vi "SingleGUI_dualCH.vi"() -> ()   [LabVIEW 8.6]
uses:
  <vilib>/event_ctls.llb/lveventtype.ctl
  <vilib>/Utility/inputDevices.llb/mouseAcquire.vi
  <vilib>/Utility/inputDevices.llb/closeMouse.vi
panel:
  in  "EPI LED 3":bool
  in  "EPI LED 2":bool
  in  "Intensity 3":dbl(slide)
  in  "Intensity 2":dbl(slide)
  in  "Menu":string
  in  "Channel1":bool
  in  "Intensity":dbl(slide)
  in  "PMT2 ON":bool caption="PMT2"
  in  "High Voltage PMT / V 2":u16(slide) caption="High Voltage PMT2 / V"
  out "Gain 2":dbl caption="Gain 1" format="%^#_4g"
  in  "Pos [mm]":cluster{"x":dbl, "y":dbl} {"x" format="%.4f"; "y" format="%.4f"}
  in  "Stage control":enum32{"xy", "Setup", "Status"}(tab)
  in  "Stepsize [mm]":dbl(slide)
  in  "Cluster":T1
  in  "clockwise":bool
  in  "xy Angle":dbl
  out "scroll units^3":dbl
  out "Mouse inside?":T2
  out "scroll timed out":bool
  out "endGUI":bool
  in  "z[mm]":dbl(slide) scale format="%#.3f"
  in  "PMT Filter":sgl(ring) caption="filter.f1" items=["Split562", "Split495", "empty"]
  in  "Epi Filter":sgl(ring) caption="filter.f2" items=["emty", "empty"]
  in  "close":bool
  in  "PMT1 ON":bool caption="PMT1"
  in  "High Voltage PMT / V":u16(slide)
  out "Gain":dbl caption="Gain 1" format="%^#_4g"
  in  "stop 2":bool
  in  "continous":bool
  in  "EPI LED":bool
  in  "single":bool
  in  "Exposure (s)":dbl(slide) scale format="%#.3p"
  out "Image":T3(plugin-control)
  in  "Detector":u16(ring)
  out "Image Number":i32
  in  "Conversion Method":u32(ring) items=["Full Dynamic", "Given Range", "90% Dynamic", "Given Percent Range"]
  in  "Maximum Value":i32
  in  "Minimum Value":i32
  # "Colibri Laser Scanning                                                                                                                                                         TILL Photonics GmbH"
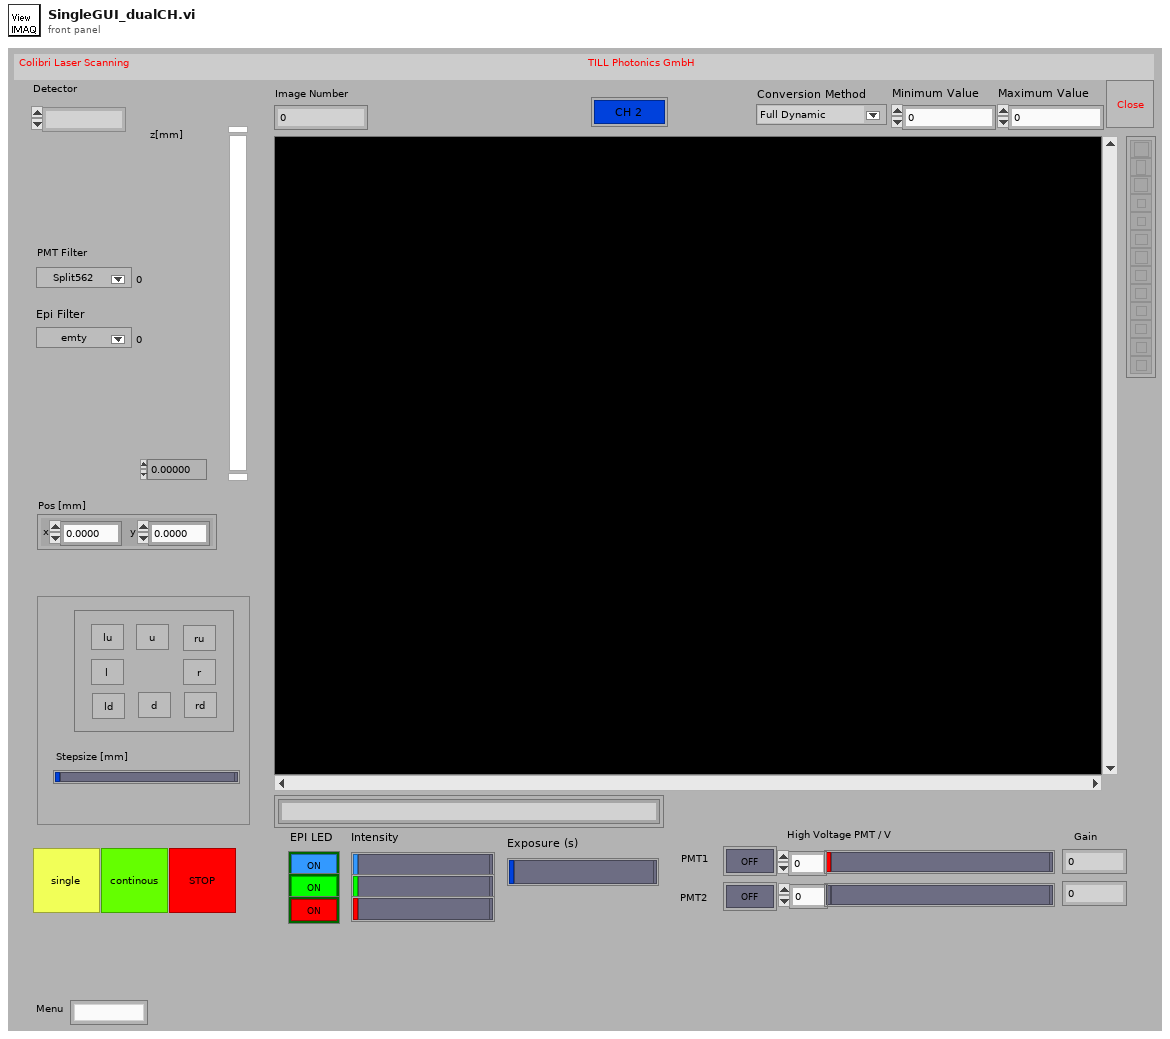
[diagram p1: front panel]
types:
  T1 = cluster{"r":bool, "ru":bool, "u":bool, "lu":bool, "l":bool, "ld":bool, "d":bool, "rd":bool}
  T2 = typedef "lveventtype.ctl" = enum32{"Null", "Timeout", "App Instance Close", "App Instance Close?", "Autoscale Range Change", "Cell Edit", "Cell Edit?", "Cursor Grab", "Cursor Grab?", "Cursor Move", "Cursor Release", "Data Change", "Direction Change", "Display State Change", "Drag Ended", "Drag Enter", "Drag Leave", "Drag Over", "Drag Source Update", "Drag Starting", "Drag Starting?", "Drop", "Exec State Change", "Key Down", "Key Down?", "Key Repeat", "Key Repeat?", "Key Up", "Listbox Double Click", "Menu Activation?", "Menu Selection (App)", "Menu Selection? (App)", "Menu Selection (User)", "Mouse Down", "Mouse Down?", "Mouse Enter", "Mouse Leave", "Mouse Move", "Mouse Up", "NI Security User Change (App)", "Pane Size", "Panel Close", "Panel Close?", "Panel Resize", "Plot Attribute Change", "Scale Range Change", "Shortcut Menu Activation?", "Shortcut Menu Selection (App)", "Shortcut Menu Selection? (App)", "Shortcut Menu Selection (User)", "Tree Double Click", "Tree Drag", "Tree Drag?", "Tree Drop", "Tree Drop?", "Tree Item Close", "Tree Item Close?", "Tree Item Open", "Tree Item Open?", "Value Change"}
  T3 = typedef "IMAQ Image.ctl" = refnum<image>
  T4 = enum16{"None/#Datasets", "Clear", "TagValueOf#", "AddValues", "ReadValue", "ChangeValue", "Get all"}
  T5 = enum16{"status", "createIMAQ", "getIMAQ", "getNumber", "deleteIMAQ", "deleteAll", "MemoryUsage", "GetAccess", "DecreaseAccess", "ActualIndex", "ElementToNumber"}
  T6 = cluster{"menu tag":string, "menu-vi":refnum<vi>}[]
  T7 = cluster{"Horizontal":i32, "Vertical":i32, "Scrolling":i32}
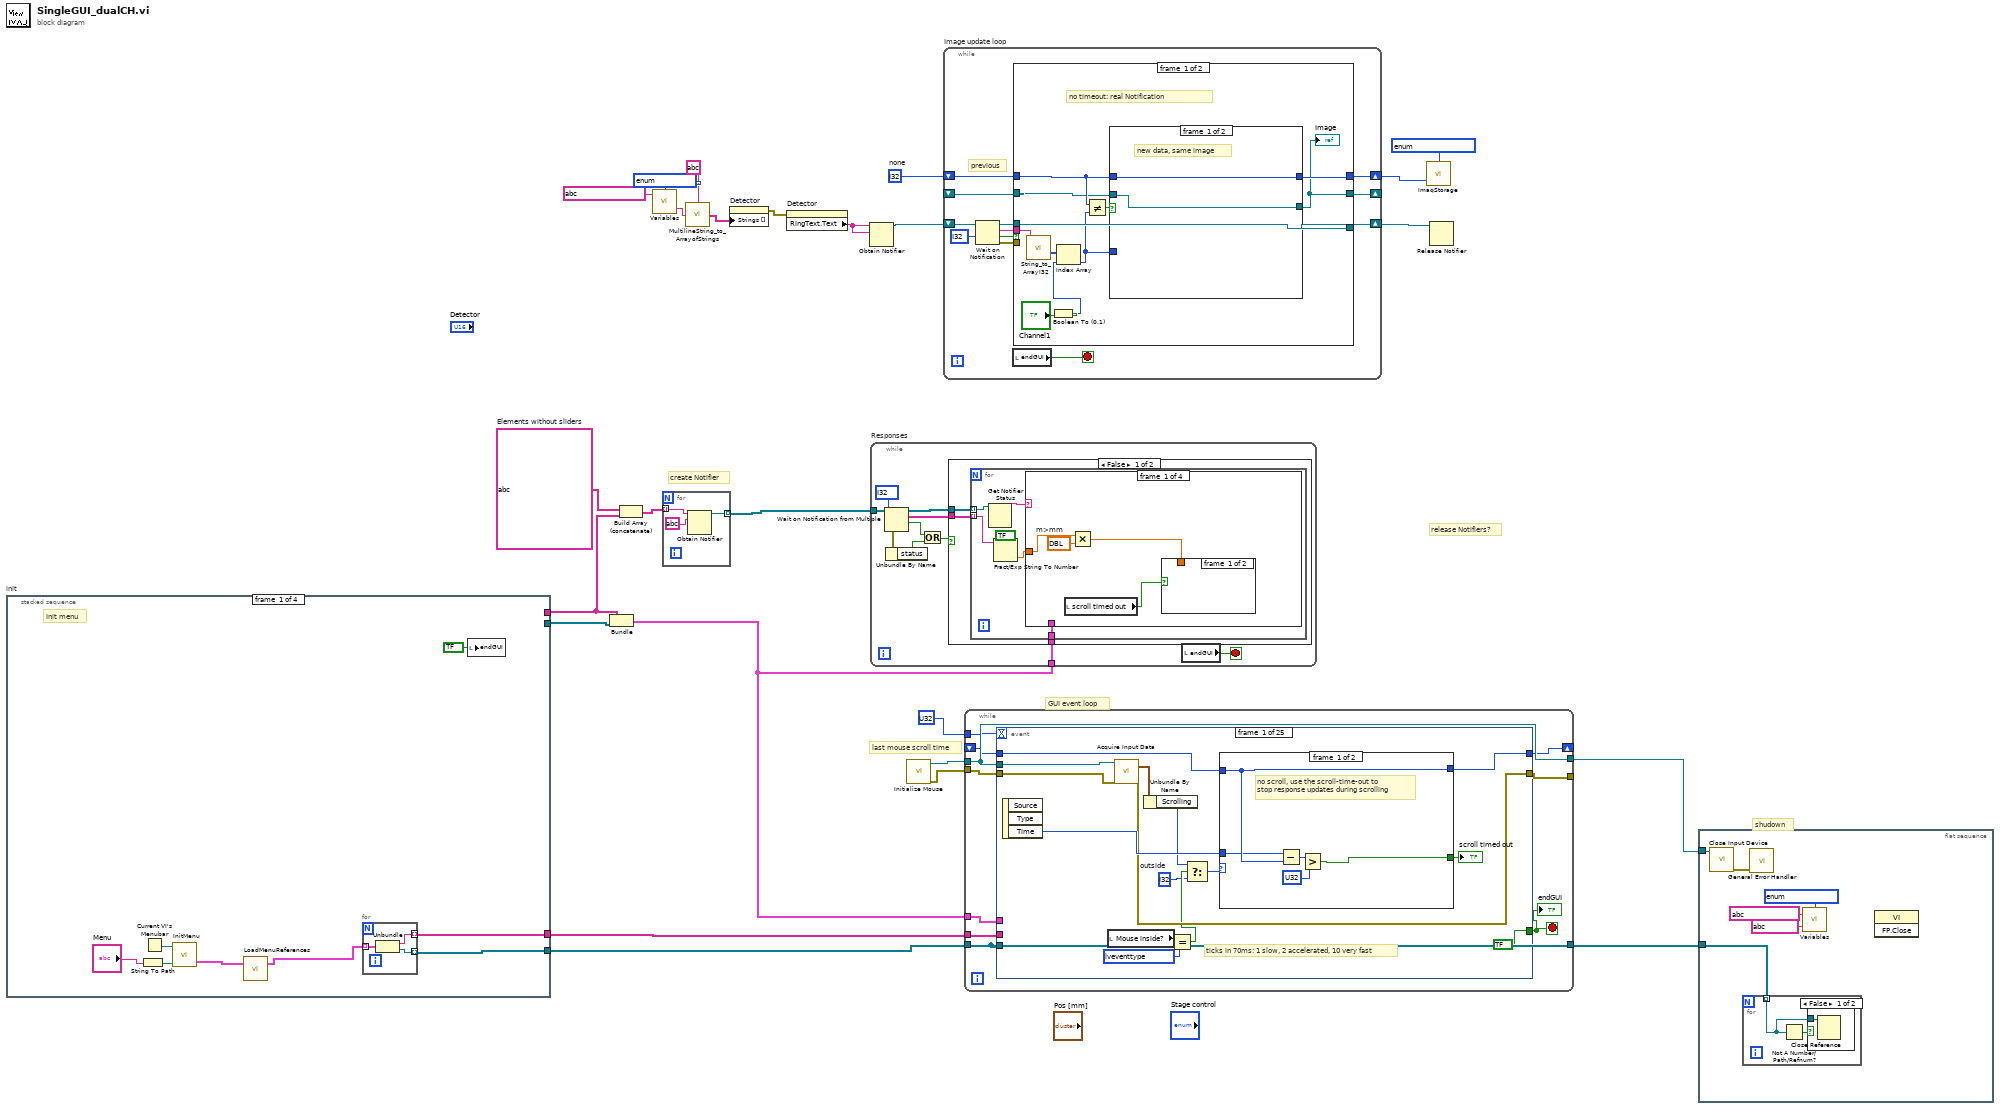
[diagram p0: block diagram]
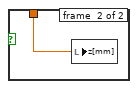
[diagram p3: hidden frame]
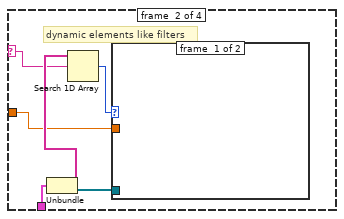
[diagram p4: hidden frame]
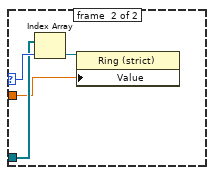
[diagram p5: hidden frame]
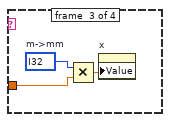
[diagram p6: hidden frame]
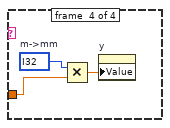
[diagram p7: hidden frame]
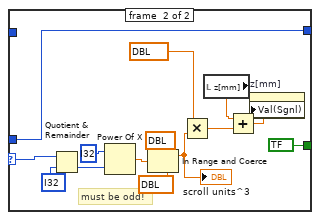
[diagram p9: hidden frame]
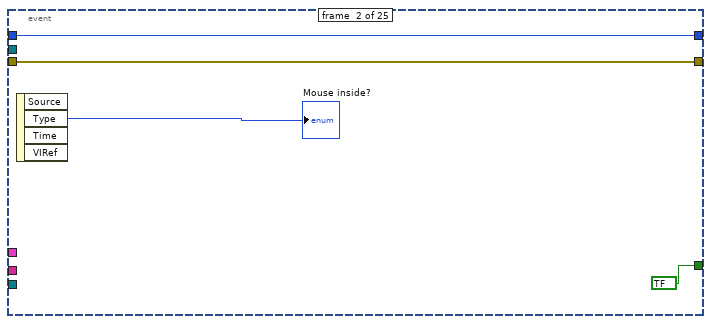
[diagram p10: hidden frame]
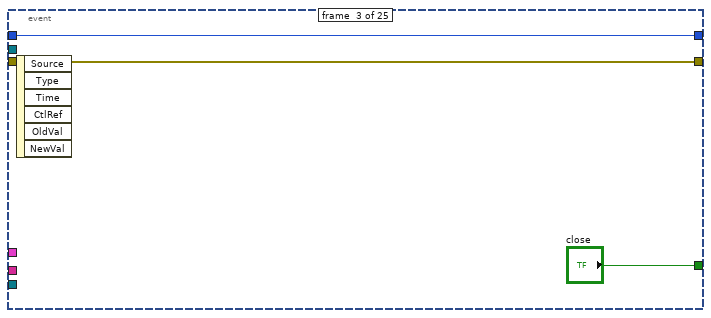
[diagram p11: hidden frame]
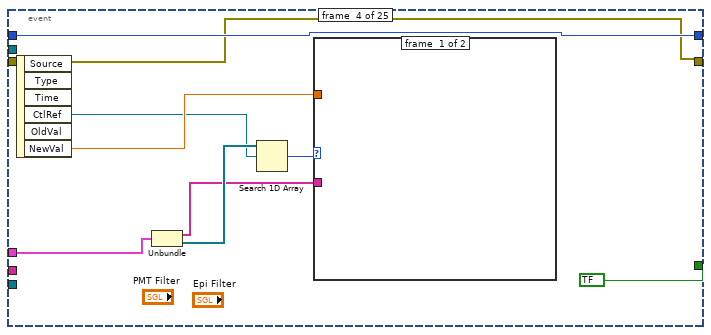
[diagram p12: hidden frame]
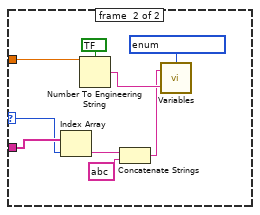
[diagram p13: hidden frame]
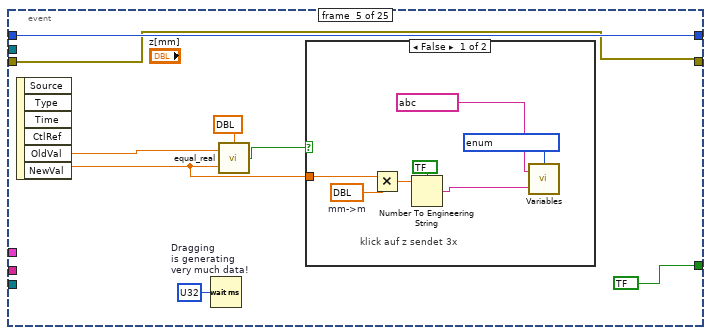
[diagram p14: hidden frame]
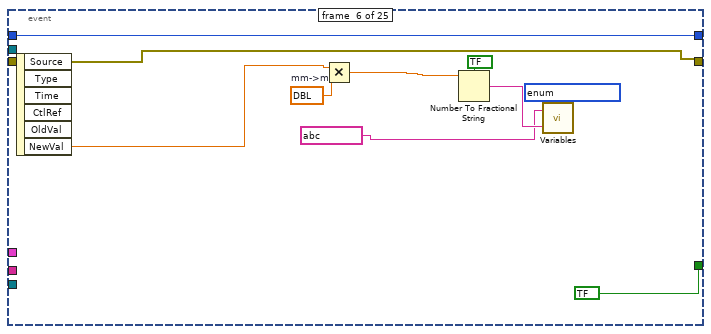
[diagram p16: hidden frame]
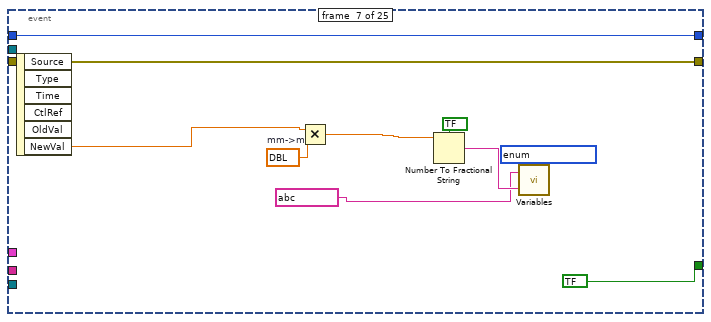
[diagram p17: hidden frame]
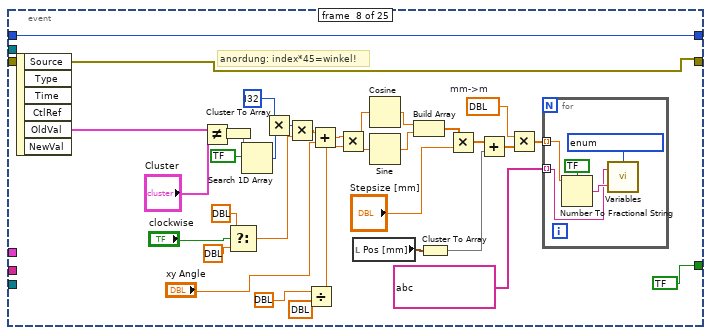
[diagram p18: hidden frame]
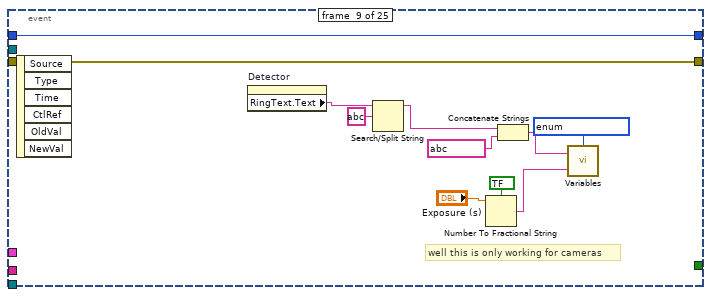
[diagram p19: hidden frame]
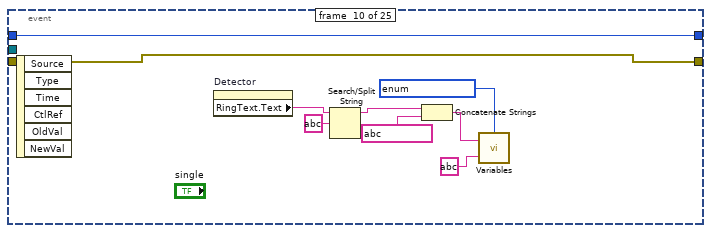
[diagram p20: hidden frame]
diagram:
  w13 = string[] ?  # Elements without sliders
  w22 = i32 ?  # none
  # "shudown"
  # "last mouse scroll time"
  # "release Notifiers?"
  # "create Notifier"
  # "GUI event loop"
  n1 = stacked-sequence "init" {
    tunnel: [_ w41 _ _] -> w11
    tunnel: [_ w40 _ _] -> w9
    tunnel: [w27 _ _ _] -> w4
    tunnel: [w26 _ _ _] -> w3
    frame #0 {
      # "Init menu"
      n2 = String To Path(string="Menu") -> (path=w30:path)
      n3 = Current VI's Menubar() -> (w32:refnum<k9>)
      n4 = call "InitMenu.vi"("menu-ini"=w30, "menubar"=w32) -> ("Menu-VI"=w31:cluster{"item tag":string, "vi-Path":path}[])  [unwired: 1 out]
      n5 = call "LoadMenuReferences.vi"("Menu-VI"=w31) -> ("Menu"=w28:T6)  [unwired: 1 in, 1 out]
      n6 = for {
        tunnel: w28 -> [w36] mode=indexing
        tunnel: [w35] -> w27 mode=indexing
        tunnel: [w34] -> w26 mode=indexing
        n7 = Unbundle(w36) -> ("menu tag"=w35:string, "menu-vi"=w34:refnum<vi>)
      }
      n8 = local write "endGUI"(bool ? ("stop 2")) -> ()
    }
    frame #1 {
      # "Init filter slider controls"
      n9 = call "Variables.vi"("Tag in"=string ?, "Command"=T4 ?) -> ("value out"=w43:string)  [unwired: 1 in, 2 out]
      n10 = call "MultilineString_to_ArrayofStrings.vi"("String 1"=w43, "NewLineString"=string ?) -> ("String Array"=w41:string[])
      n11 = control-ref of="Epi Filter"() -> (w39:refnum<vi>)
      n12 = control-ref of="PMT Filter"() -> (w38:refnum<vi>)
      n13 = Build Array(w38, w39) -> (w37:refnum<vi>[])
      n14 = for {
        tunnel: w41 -> [w49] mode=indexing
        tunnel: w37 -> [w47] mode=indexing
        tunnel: [w46] -> w40 mode=indexing
        n15 = Concatenate Strings(w49, string ? ("string")) -> (w50:string)
        n16 = call "Variables.vi"("Tag in"=w50, "Command"=T4 ?) -> ("value out"=w54:string)  [unwired: 1 in, 2 out]
        n17 = call "MultilineString_to_ArrayofStrings.vi"("String 1"=w54, "NewLineString"=string ?) -> ("String Array"=w53:string[])
        n18 = for {
          tunnel: w53 -> [w63] mode=indexing
          tunnel: [w58] -> w52 mode=indexing
          n19 = call "SplitAtLast.vi"("search char"=string ?, "In-String"=w63) -> ("end"=w61:string, "Front (default)"=w60:string)
          n20 = Fract/Exp String To Number(use system decimal point (T)=bool ?, string=w61) -> (number=w59:dbl)  [unwired: 3 out]
          n21 = Bundle("Front (default)"=w60, w59) -> (w58:cluster{"Front (default)":string, dbl})  [unwired: 1 out]
        }
        n22 = property on="Property Node" class="Ring (strict)"(reference=w47, "StringsAndValues[]"=w52, "Visible"=bool ?, "Caption.Text"=w49) -> (reference out=w46:refnum<vi>)  [unwired: 1 in, 1 out]
      }
    }
    frame #2 {
      # "it would be good to Read/update all elements\nbut this is usually done by \"update\" to the .set variables after the return Notifiers are listening\nhere just z is updated"
      n23 = call "Variables.vi"("Tag in"=string ?, "Command"=T4 ?) -> ("value out"=w67:string)  [unwired: 1 in, 2 out]
      n24 = Fract/Exp String To Number(use system decimal point (T)=bool ?, string=w67) -> (number=w66:dbl)  [unwired: 3 out]
      n25 = Multiply(x=dbl ?, y=w66) -> (x*y=w65:dbl)
      n26 = local write "z[mm]"(w65) -> ()
    }
    frame #3 {
      n27 = property on="Image" class="ImageControl"() -> ("16-bit Display Conversion Method"=w71:u32)  [unwired: 2 in, 2 out]
      n28 = local write "Conversion Method"(w71) -> ()
    }
  }
  n29 = Bundle("String Array"=w11, w9) -> (w10:cluster{"String Array":string[], refnum<vi>[]})  [unwired: 1 out]
  n30 = Build Array (concatenate)(w13, w11) -> (w12:string[])
  n31 = call "Variables.vi"("Tag in"=string ?, "Command"=T4 ?) -> ("value out"=w17:string)  [unwired: 1 in, 2 out]
  n32 = for {
    tunnel: w12 -> [w73] mode=indexing
    tunnel: [w74] -> w8 mode=indexing
    n33 = Obtain Notifier(name (unnamed)=w73, notification data type=string ?) -> (notifier out=w74:refnum<notifier>)  [unwired: 2 in, 2 out]
  }
  n34 = call "MultilineString_to_ArrayofStrings.vi"("String 1"=w17, "NewLineString"=string ?) -> ("String Array"=w15:string[])
  n35 = property on="Detector" class="Ring (strict)"("Strings []"=w15) -> (error out=w14:errorcluster)  [unwired: 2 in, 1 out]
  n36 = property on="Detector" class="Ring (strict)"(error in=w14) -> ("RingText.Text"=w23:string)  [unwired: 1 in, 2 out]
  n37 = Obtain Notifier(name (unnamed)=w23, notification data type=w23) -> (notifier out=w25:refnum<notifier>)  [unwired: 2 in, 2 out]
  n38 = while "Responses" {
    tunnel: w8 -> [w84]
    tunnel: w10 -> [w76]
    stop <- w75 stop-if-true
    n39 = Wait on Notification from Multiple(0:w84, 2:i32 ? ("timeout in ms (-1)")) -> (8:w79:refnum<notifier>[], 9:w78:string[], 10:w80:bool, 11:w82:errorcluster)  [unwired: 1 in, 1 out]
    n40 = Unbundle By Name(w82) -> ("status"=w81:bool)
    n41 = Or(x=w80, y=w81) -> (x .or. y?=w77:bool)
    n42 = case shown="False" w77 {
      tunnel: w79 -> [w87 _]
      tunnel: w78 -> [w86 _]
      tunnel: w76 -> [w85 _]
      frame #0 {
        n43 = for {
          tunnel: w87 -> [w93] mode=indexing
          tunnel: w86 -> [w91] mode=indexing
          tunnel: w85 -> [w88]
          n44 = Get Notifier Status(notifier=w93) -> (notifier name=w92:string)  [unwired: 1 in, 4 out]
          n45 = Fract/Exp String To Number(use system decimal point (T)=bool ?, string=w91) -> (number=w89:dbl)  [unwired: 3 out]
          n46 = case shown="\"filter.f1\", Default" w92 {
            selector: w92 -> [_ w101 _ _]
            tunnel: w89 -> [w97 w99 w110 w114]
            tunnel: w88 -> [_ w104 _ _]
            frame #0 {
              w95 = dbl ?  # m>mm
              n47 = local read "scroll timed out"() -> (w94:bool)
              n48 = Multiply(x=w97, y=w95) -> (x*y=w96:dbl)
              n49 = case shown="True" w94 {
                tunnel: w96 -> [_ w98]
                frame #0 {
                }
                frame #1 {
                  n50 = local write "z[mm]"(w98) -> ()
                }
              }
            }
            frame #1 {
              # "dynamic elements like filters"
              n51 = Unbundle(w104) -> ("String Array"=w102:string[], w103:refnum<vi>[])
              n52 = Search 1D Array(1D array=w102, element=w101) -> (index of element=w100:i32)  [unwired: 1 out]
              n53 = case shown="0.." w100 {
                selector: w100 -> [_ w108]
                tunnel: w103 -> [_ w107]
                tunnel: w99 -> [_ w105]
                frame #0 {
                }
                frame #1 {
                  n54 = Index Array(array=w107, index=w108) -> (element=w106:refnum<vi>)
                  n55 = property on="Property Node" class="Ring (strict)"(reference=w106, "Value"=w105) -> ()  [unwired: 1 in, 2 out]
                }
              }
            }
            frame #2 {
              w111 = i32 ?  # m->mm
              n56 = Multiply(x=w111, y=w110) -> (x*y=w109:dbl)
              n57 = property on="x" class="DigNum (strict)"("Value"=w109) -> ()  [unwired: 2 in, 2 out]
            }
            frame #3 {
              w113 = i32 ?  # m->mm
              n58 = Multiply(x=w113, y=w114) -> (x*y=w112:dbl)
              n59 = property on="y" class="DigNum (strict)"("Value"=w112) -> ()  [unwired: 2 in, 2 out]
            }
          }
        }
      }
      frame #1 {
        # "err or timeout"
      }
    }
    n60 = local read "endGUI"() -> (w75:bool)
  }
  n61 = call <vilib>:"Initialize Mouse.vi"() -> ("error out"=w6:errorcluster, "device ID"=w7:refnum<k1>)  [unwired: 1 in, 9 out]
  n62 = while "Image update loop" {
    shift-right: [w124] -> w21
    shift-left: w22 -> [w125]
    shift-right: [w119] -> w24
    shift-left: w25 -> [w126]
    shift-right: [w118] -> _
    shift-left: _ -> [w117]
    stop <- w116 stop-if-true
    # "previous"
    n63 = Wait on Notification(notifier=w126, timeout in ms (-1)=i32 ?) -> (notifier out=w120:refnum<notifier>, notification=w115:string, timed out?=w122:bool, error out=w123:errorcluster)  [unwired: 1 in, 1 out]
    n64 = local read "endGUI"() -> (w116:bool)
    n65 = case shown="True" w122 {
      tunnel: w115 -> [w131 _]
      tunnel: w125 -> [w136 w152]
      tunnel: [w133 w152] -> w124
      tunnel: w123 -> [_ _]
      tunnel: w120 -> [w137 w151]
      tunnel: [w137 w147] -> w119
      tunnel: [w132 w145] -> w118
      tunnel: w117 -> [w134 w145]
      frame #0 {
        # "no timeout: real Notification"
        n66 = call "String_to_ArrayI32.vi"("String"=w131) -> ("ArrayI32"=w130:i32[])  [unwired: 1 in]
        n67 = Boolean To (0,1)(Boolean="Channel1") -> (0, 1=w127:i16)
        n68 = Index Array(array=w130, index=w127) -> (element=w129:i32)
        n69 = Not Equal?(x=w136, y=w129) -> (x != y?=w135:bool)
        n70 = case shown="True" w135 {
          tunnel: [w139 w144] -> w132
          tunnel: w129 -> [_ w140]
          tunnel: w136 -> [w138 w143]
          tunnel: w134 -> [w139 _]
          tunnel: [w138 w140] -> w133
          frame #0 {
            # "new data, same image"
          }
          frame #1 {
            # "only valid if\nstill in memory!"
            # "new image"
            n71 = call "ImaqStorage.vi"("Number"=w143, "Command"=T5 ?) -> ()  [unwired: 1 in, 2 out]
            n72 = call "ImaqStorage.vi"("Number"=w140, "Command"=T5 ?) -> ("IMAQ out"=w144:T3)  [unwired: 1 in, 1 out]
            "Image Number" <- w140
          }
        }
        "Image" <- w132
      }
      frame #1 {
        # "time out\ngood for checking the stop button\nis there a new detektor?"
        n73 = property on="Detector" class="Ring (strict)"() -> ("RingText.Text"=w146:string)  [unwired: 2 in, 2 out]
        n74 = Get Notifier Status(notifier=w151) -> (notifier out=w148:refnum<notifier>, notifier name=w150:string)  [unwired: 1 in, 3 out]
        n75 = Not Equal?(x=w146, y=w150) -> (x != y?=w149:bool)
        n76 = case shown="True" w149 {
          tunnel: w148 -> [w153 w156]
          tunnel: [w153 w155] -> w147
          tunnel: w146 -> [_ w154]
          frame #0 {
            # "same as before"
          }
          frame #1 {
            n77 = Release Notifier(notifier=w156) -> ()  [unwired: 1 in, 4 out]
            n78 = Obtain Notifier(name (unnamed)=w154, notification data type=w154) -> (notifier out=w155:refnum<notifier>)  [unwired: 2 in, 2 out]
          }
        }
      }
    }
  }
  n79 = while {
    tunnel: w10 -> [w166]
    tunnel: w7 -> [w165]
    tunnel: [w165] -> w2
    tunnel: w6 -> [w164]
    tunnel: [w163] -> _
    shift-right: [w161] -> _
    shift-left: _ -> [w162]
    tunnel: u32 ? ("milliseconds to wait") -> [w159]
    tunnel: w4 -> [w158]
    tunnel: w3 -> [w157]
    tunnel: [w157] -> w1
    stop <- w160 stop-if-true
    n80 = event shown="[23] Menu Selection (User)" {
      selector: _ -> [_ _ _ _ _ _ _ _ _ _ _ _ _ _ _ _ _ _ _ _ _ _ _ _ _]
      dyn-events: _ -> [_ _ _ _ _ _ _ _ _ _ _ _ _ _ _ _ _ _ _ _ _ _ _ _ _]
      timeout: w159 -> [_ _ _ _ _ _ _ _ _ _ _ _ _ _ _ _ _ _ _ _ _ _ _ _ _]
      tunnel: [bool ? ("stop") bool ? ("stop") "close" bool ? bool ? bool ? bool ? ("stop") bool ? ("stop") _ _ _ _ _ _ _ _ _ _ bool ? ("stop") bool ? ("stop") _ _ _ w432 w445] -> w160
      tunnel: w166 -> [_ _ _ w214 _ _ _ _ _ _ _ _ _ _ _ _ _ _ _ _ _ _ _ _ _]
      tunnel: w165 -> [w181 _ _ _ _ _ _ _ _ _ _ _ _ _ _ _ _ _ _ _ _ _ _ _ _]
      tunnel: w164 -> [w180 w201 w205 w208 w226 w242 w251 w261 w302 w313 w319 w327 w335 w346 w355 w361 w366 w375 w385 w397 w410 w417 w424 _ _]
      tunnel: [w173 w201 w205 w208 w226 w242 w251 w261 w302 w313 w319 w327 w335 w346 w355 w361 w366 w375 w385 w397 w410 w417 w424 _ _] -> w163
      tunnel: w162 -> [w177 w202 w206 w209 w227 w241 w252 w262 w303 w314 w320 w328 w336 w347 w356 w362 w367 w376 w386 w398 w416 w423 w430 w431 w444]
      tunnel: [w178 w202 w206 w209 w227 w241 w252 w262 w303 w314 w320 w328 w336 w347 w356 w362 w367 w376 w386 w398 w416 w423 w430 w431 w444] -> w161
      tunnel: w158 -> [_ _ _ _ _ _ _ _ _ _ _ _ _ _ _ _ _ _ _ _ _ _ _ w434 _]
      tunnel: w157 -> [_ _ _ _ _ _ _ _ _ _ _ _ _ _ _ _ _ _ _ _ _ _ _ w433 _]
      event #0 {
        w167 = i32 ?  # outside
        # "ticks in 70ms: 1 slow, 2 accelerated, 10 very fast"
        n81 = event-data() -> ("Time"=w176:u32)  [unwired: 3 out]
        n82 = local read "Mouse inside?"() -> (w172:T2)
        n83 = call-poly <vilib>:"Acquire Input Data.vi"("device ID"=w181, "error in (no error)"=w180) -> ("axis info"=w179:T7, "error out"=w173:errorcluster)  [unwired: 1 in, 15 out]
        n84 = Unbundle By Name(w179) -> ("Scrolling"=w169:i32)
        n85 = Equal?(x=w172, y=T2 ? ("Type")) -> (x = y?=w170:bool)
        n86 = Select(t=w169, s=w170, f=w167) -> (s? t:f=w168:i32)
        n87 = case shown="1, Default" w168 {
          selector: w168 -> [_ w196]
          tunnel: w177 -> [w186 _]
          tunnel: [w186 w197] -> w178
          tunnel: w176 -> [w183 w197]
          tunnel: [w182 bool ?] -> w174
          frame #0 {
            # "no scroll, use the scroll-time-out to\nstop response updates during scrolling"
            n88 = Subtract(x=w183, y=w186) -> (x-y=w185:u32)
            n89 = Greater?(x=w185, y=u32 ?) -> (0:w182:bool)
          }
          frame #1 {
            # "must be odd!"
            n90 = Quotient & Remainder(x=w196, y=i32 ?) -> (floor(x/y)=w194:i32)  [unwired: 1 out]
            n91 = Power Of X(1:w194, 2:i32 ? ("y")) -> (0:w192:dbl)
            n92 = In Range and Coerce(upper limit=dbl ?, x=w192, lower limit=dbl ?) -> (coerced(x)=w191:dbl)  [unwired: 1 out]
            "scroll units^3" <- w191
            n93 = Multiply(x=dbl ? ("min.step"), y=w191) -> (x*y=w200:dbl)
            n94 = local read "z[mm]"() -> (w199:dbl)
            n95 = Add(x=w199, y=w200) -> (x+y=w198:dbl)
            n96 = property on="z[mm]" class="Slide (strict)"("Val(Sgnl)"=w198) -> ()  [unwired: 2 in, 2 out]
          }
        }
        "scroll timed out" <- w174
      }
      event #1 {
        n97 = event-data() -> ("Type"=→"Mouse inside?":T2)  [unwired: 4 out]
      }
      event #2 {
        n98 = event-data() -> ()  [unwired: 7 out]
      }
      event #3 {
        n99 = event-data() -> ("CtlRef"=w212:refnum<vi>, "NewVal"=w216:sgl)  [unwired: 5 out]
        n100 = Unbundle(w214) -> ("String Array"=w210:string[], w213:refnum<vi>[])
        n101 = Search 1D Array(1D array=w213, element=w212) -> (index of element=w211:i32)  [unwired: 1 out]
        n102 = case shown="0.." w211 {
          selector: w211 -> [_ w220]
          tunnel: w216 -> [_ w225]
          tunnel: w210 -> [_ w221]
          frame #0 {
          }
          frame #1 {
            n103 = Index Array(array=w221, index=w220) -> (element=w219:string)
            n104 = Number To Engineering String(1:bool ? ("use system decimal point (T)"), 4:w225) -> (0:w224:string)  [unwired: 2 out]
            n105 = Concatenate Strings(w219, string ? ("string")) -> (w218:string)
            n106 = call "Variables.vi"("value"=w224, "Tag in"=w218, "Command"=T4 ?) -> ()  [unwired: 3 out]
          }
        }
      }
      event #4 {
        w232 = u32 ?  # Dragging is generating very much data!
        n107 = event-data() -> ("OldVal"=w231:dbl, "NewVal"=w230:dbl)  [unwired: 5 out]
        n108 = Wait (ms)(milliseconds to wait=w232) -> ()  [unwired: 1 out]
        n109 = call "equal_real.vi"("max rel deviation"=dbl ?, "b"=w230, "a"=w231) -> ("Equal"=w229:bool)
        n110 = case shown="False" w229 {
          tunnel: w230 -> [w235 _]
          frame #0 {
            w240 = dbl ?  # mm->m
            # "klick auf z sendet 3x"
            n111 = Multiply(x=w235, y=w240) -> (x*y=w239:dbl)
            n112 = Number To Engineering String(1:bool ? ("use system decimal point (T)"), 4:w239) -> (0:w237:string)  [unwired: 2 out]
            n113 = call "Variables.vi"("value"=w237, "Tag in"=string ?, "Command"=T4 ?) -> ()  [unwired: 3 out]
          }
          frame #1 {
          }
        }
      }
      event #5 {
        w249 = dbl ?  # mm->m
        n114 = event-data() -> ("NewVal"=w247:dbl)  [unwired: 6 out]
        n115 = Multiply(x=w247, y=w249) -> (x*y=w250:dbl)
        n116 = Number To Fractional String(use system decimal point (T)=bool ?, number=w250) -> (F-format string=w245:string)  [unwired: 2 out]
        n117 = call "Variables.vi"("value"=w245, "Tag in"=string ? ("Tag"), "Command"=T4 ?) -> ()  [unwired: 3 out]
      }
      event #6 {
        w259 = dbl ?  # mm->m
        n118 = event-data() -> ("NewVal"=w254:dbl)  [unwired: 6 out]
        n119 = Multiply(x=w254, y=w259) -> (x*y=w260:dbl)
        n120 = Number To Fractional String(use system decimal point (T)=bool ?, number=w260) -> (F-format string=w257:string)  [unwired: 2 out]
        n121 = call "Variables.vi"("value"=w257, "Tag in"=string ? ("Tag"), "Command"=T4 ?) -> ()  [unwired: 3 out]
      }
      event #7 {
        w277 = dbl ?  # mm->m
        # "anordung: index*45=winkel!"
        n122 = event-data() -> ("OldVal"=w293:T1)  [unwired: 6 out]
        n123 = Not Equal?(x=w293, y="Cluster") -> (x != y?=w292:T1)
        n124 = Cluster To Array(cluster=w292) -> (array=w291:bool[])
        n125 = Select(t=dbl ?, s="clockwise", f=dbl ?) -> (s? t:f=w266:dbl)
        n126 = Search 1D Array(1D array=w291, element=bool ? ("Element")) -> (index of element=w289:i32)  [unwired: 1 out]
        n127 = Multiply(x=i32 ?, y=w289) -> (x*y=w288:i32)
        n128 = Multiply(x=w288, y=w266) -> (x*y=w267:dbl)
        n129 = Divide(x=dbl ?, y=dbl ?) -> (x/y=w268:dbl)
        n130 = Add(x=w267, y="xy Angle") -> (x+y=w265:dbl)
        n131 = Multiply(x=w265, y=w268) -> (x*y=w275:dbl)
        n132 = local read "Pos [mm]"() -> (w282:cluster{"x":dbl, "y":dbl})
        n133 = Cosine(x=w275) -> (cos(x)=w285:dbl)
        n134 = Sine(x=w275) -> (sin(x)=w284:dbl)
        n135 = Build Array(w285, w284) -> (w283:dbl[])
        n136 = Cluster To Array(cluster=w282) -> (array=w281:dbl[])
        n137 = Multiply(x=w283, y="Stepsize [mm]") -> (x*y=w286:dbl[])
        n138 = Add(x=w286, y=w281) -> (x+y=w279:dbl[])
        n139 = Multiply(x=w277, y=w279) -> (x*y=w278:dbl[])
        n140 = for {
          tunnel: w278 -> [w294] mode=indexing
          tunnel: string[] ? -> [w295] mode=indexing
          n141 = Number To Fractional String(use system decimal point (T)=bool ?, number=w294) -> (F-format string=w298:string)  [unwired: 2 out]
          n142 = call "Variables.vi"("value"=w298, "Tag in"=w295, "Command"=T4 ?) -> ()  [unwired: 3 out]
        }
      }
      event #8 {
        # "well this is only working for cameras"
        n143 = event-data() -> ()  [unwired: 7 out]
        n144 = property on="Detector" class="Ring (strict)"() -> ("RingText.Text"=w300:string)  [unwired: 2 in, 2 out]
        n145 = Search/Split String(string=w300, search string/char (-)=string ? ("Nach String/Zeichen suchen (-)")) -> (substring before match=w299:string)  [unwired: 3 out]
        n146 = Number To Fractional String(use system decimal point (T)=bool ?, number="Exposure (s)") -> (F-format string=w306:string)  [unwired: 2 out]
        n147 = Concatenate Strings(w299, string ? ("Tag in")) -> (w309:string)
        n148 = call "Variables.vi"("value"=w306, "Tag in"=w309, "Command"=T4 ?) -> ()  [unwired: 3 out]
      }
      event #9 {
        n149 = event-data() -> ()  [unwired: 7 out]
        n150 = property on="Detector" class="Ring (strict)"() -> ("RingText.Text"=w311:string)  [unwired: 2 in, 2 out]
        n151 = Search/Split String(string=w311, search string/char (-)=string ? ("Nach String/Zeichen suchen (-)")) -> (substring before match=w310:string)  [unwired: 3 out]
        n152 = Concatenate Strings(w310, string ? ("notification")) -> (w317:string)
        n153 = call "Variables.vi"("value"=string ? ("notification"), "Tag in"=w317, "Command"=T4 ?) -> ()  [unwired: 3 out]
      }
      event #10 {
        n154 = event-data() -> ()  [unwired: 7 out]
        n155 = Select(t=string ? ("value"), s="EPI LED", f=string ?) -> (s? t:f=w325:string)
        n156 = call "Variables.vi"("value"=w325, "Tag in"=string ?, "Command"=T4 ?) -> ()  [unwired: 3 out]
      }
      event #11 {
        n157 = event-data() -> ()  [unwired: 7 out]
        n158 = Select(t=string ? ("value"), s="EPI LED 3", f=string ?) -> (s? t:f=w333:string)
        n159 = call "Variables.vi"("value"=w333, "Tag in"=string ?, "Command"=T4 ?) -> ()  [unwired: 3 out]
      }
      event #12 {
        n160 = event-data() -> ()  [unwired: 7 out]
        n161 = Select(t=string ? ("value"), s="EPI LED 2", f=string ?) -> (s? t:f=w341:string)
        n162 = call "Variables.vi"("value"=w341, "Tag in"=string ?, "Command"=T4 ?) -> ()  [unwired: 3 out]
      }
      event #13 {
        n163 = event-data() -> ()  [unwired: 7 out]
        n164 = property on="Detector" class="Ring (strict)"() -> ("RingText.Text"=w344:string)  [unwired: 2 in, 2 out]
        n165 = Search/Split String(string=w344, search string/char (-)=string ? ("Nach String/Zeichen suchen (-)")) -> (substring before match=w343:string)  [unwired: 3 out]
        n166 = Concatenate Strings(w343, string ? ("notification")) -> (w351:string)
        n167 = call "Variables.vi"("value"=string ? ("notification"), "Tag in"=w351, "Command"=T4 ?) -> ()  [unwired: 3 out]
      }
      event #14 {
        n168 = event-data() -> ()  [unwired: 7 out]
        n169 = property on="Detector" class="Ring (strict)"() -> ("RingText.Text"=w353:string)  [unwired: 2 in, 2 out]
        n170 = Search/Split String(string=w353, search string/char (-)=string ? ("Nach String/Zeichen suchen (-)")) -> (substring before match=w352:string)  [unwired: 3 out]
        n171 = Concatenate Strings(w352, string ? ("notification")) -> (w359:string)
        n172 = call "Variables.vi"("value"=string ? ("notification"), "Tag in"=w359, "Command"=T4 ?) -> ()  [unwired: 3 out]
      }
      event #15 {
        n173 = event-data() -> ()  [unwired: 7 out]
        n174 = property on="Image" class="ImageControl"("16-bit Display Conversion Method"="Conversion Method", "16-bit Display Maximum Value"="Maximum Value", "16-bit Display Minimum Value"="Minimum Value") -> ()  [unwired: 2 in, 2 out]
      }
      event #16 {
        n175 = event-data() -> ("NewVal"=w368:u16)  [unwired: 6 out]
        n176 = call "PMT-Gain.vi"("Volt"=w368) -> ("Gain"=→"Gain":dbl)
        n177 = local read "PMT1 ON"() -> (w369:bool)
        n178 = case shown="True" w369 {
          tunnel: w368 -> [_ w374]
          frame #0 {
          }
          frame #1 {
            n179 = Number To Decimal String(number=w374) -> (decimal integer string=w371:string)  [unwired: 1 out]
            n180 = call "Variables.vi"("value"=w371, "Tag in"=string ?, "Command"=T4 ?) -> ()  [unwired: 3 out]
          }
        }
      }
      event #17 {
        n181 = event-data() -> ("NewVal"=w377:u16)  [unwired: 6 out]
        n182 = call "PMT-Gain.vi"("Volt"=w377) -> ("Gain"=→"Gain 2":dbl)
        n183 = local read "PMT2 ON"() -> (w378:bool)
        n184 = case shown="True" w378 {
          tunnel: w377 -> [_ w383]
          frame #0 {
          }
          frame #1 {
            n185 = Number To Decimal String(number=w383) -> (decimal integer string=w380:string)  [unwired: 1 out]
            n186 = call "Variables.vi"("value"=w380, "Tag in"=string ?, "Command"=T4 ?) -> ()  [unwired: 3 out]
          }
        }
      }
      event #18 {
        n187 = event-data() -> ()  [unwired: 7 out]
        n188 = case shown="True" "PMT1 ON" {
          tunnel: [string ? w395] -> w390
          tunnel: [u8 ? ("Disabled") u8 ? ("Disabled")] -> w391
          frame #0 {
            # "send 0"
          }
          frame #1 {
            # "send"
            n189 = Number To Decimal String(number="High Voltage PMT / V") -> (decimal integer string=w395:string)  [unwired: 1 out]
          }
        }
        n190 = property on="High Voltage PMT / V" class="Slide (strict)"("Fill Style"=w391) -> ()  [unwired: 2 in, 2 out]
        n191 = call "Variables.vi"("value"=w390, "Tag in"=string ?, "Command"=T4 ?) -> ()  [unwired: 3 out]
      }
      event #19 {
        n192 = event-data() -> ()  [unwired: 7 out]
        n193 = case shown="True" "PMT2 ON" {
          tunnel: [string ? w408] -> w403
          tunnel: [u8 ? ("Disabled") u8 ? ("Disabled")] -> w404
          frame #0 {
            # "send 0"
          }
          frame #1 {
            # "send"
            n194 = Number To Decimal String(number="High Voltage PMT / V 2") -> (decimal integer string=w408:string)  [unwired: 1 out]
          }
        }
        n195 = property on="High Voltage PMT / V 2" class="Slide (strict)"("Fill Style"=w404) -> ()  [unwired: 2 in, 2 out]
        n196 = call "Variables.vi"("value"=w403, "Tag in"=string ?, "Command"=T4 ?) -> ()  [unwired: 3 out]
      }
      event #20 {
        n197 = event-data() -> ()  [unwired: 7 out]
        n198 = Number To Fractional String(use system decimal point (T)=bool ? ("Systemdezimalzeichen verwenden (T)"), number="Intensity") -> (F-format string=w412:string)  [unwired: 2 out]
        n199 = call "Variables.vi"("value"=w412, "Tag in"=string ?, "Command"=T4 ?) -> ()  [unwired: 3 out]
      }
      event #21 {
        n200 = event-data() -> ()  [unwired: 7 out]
        n201 = Number To Fractional String(use system decimal point (T)=bool ? ("Systemdezimalzeichen verwenden (T)"), number="Intensity 2") -> (F-format string=w419:string)  [unwired: 2 out]
        n202 = call "Variables.vi"("value"=w419, "Tag in"=string ?, "Command"=T4 ?) -> ()  [unwired: 3 out]
      }
      event #22 {
        n203 = event-data() -> ()  [unwired: 7 out]
        n204 = Number To Fractional String(use system decimal point (T)=bool ? ("Systemdezimalzeichen verwenden (T)"), number="Intensity 3") -> (F-format string=w426:string)  [unwired: 2 out]
        n205 = call "Variables.vi"("value"=w426, "Tag in"=string ?, "Command"=T4 ?) -> ()  [unwired: 3 out]
      }
      event #23 {
        # "run menu"
        n206 = event-data() -> ("ItemTag"=w435:string)  [unwired: 7 out]
        n207 = Search 1D Array(1D array=w434, element=w435) -> (index of element=w436:i32)  [unwired: 1 out]
        n208 = Index Array(array=w433, index=w436) -> (element=w437:refnum<vi>)
        n209 = case shown="\"Exit\"" w435 {
          tunnel: [bool ? bool ? bool ?] -> w432
          frame #0 {
            # "no special command"
          }
          frame #1 {
          }
          frame #2 {
            n210 = call "Cancel.vi"() -> ()  [unwired: 1 out]
          }
        }
        n211 = Not A Number/Path/Refnum?(number/path/refnum=w437) -> (NaN/Path/Refnum?=w438:bool)
        n212 = case shown="False" w438 {
          tunnel: w437 -> [w443 _]
          tunnel: w435 -> [w442 _]
          frame #0 {
            n213 = call "OpenRunGUI.vi"("VI Refnum"=w443, "Menu"=w442) -> ()  [unwired: 1 out]
          }
          frame #1 {
            # "no vi defined\ne.g top level menu"
          }
        }
      }
      event #24 {
        w445 = bool ? ("Discard?")
        # "do a nice shutdown, \nclose a bit later"
        n214 = event-data() -> ()  [unwired: 5 out]
        n215 = event-data("Discard?"=w445) -> ()  [unwired: 1 in, 1 out]
      }
    }
    "endGUI" <- w160
  }
  n216 = call "ImaqStorage.vi"("Number"=w21, "Command"=T5 ?) -> ()  [unwired: 1 in, 2 out]
  n217 = Release Notifier(notifier=w24) -> ()  [unwired: 1 in, 4 out]
  n218 = flat-sequence {
    tunnel: w2 -> [w450]
    tunnel: w1 -> [w446]
    frame #0 {
      n219 = call-poly <vilib>:"Close Input Device.vi"("device ID"=w450) -> ("error out"=w451:errorcluster)  [unwired: 1 in, 8 out]
      n220 = for {
        tunnel: w446 -> [w452] mode=indexing
        n221 = Not A Number/Path/Refnum?(number/path/refnum=w452) -> (NaN/Path/Refnum?=w453:bool)
        n222 = case shown="False" w453 {
          tunnel: w452 -> [w454 _]
          frame #0 {
            n223 = Close Reference(reference=w454) -> ()  [unwired: 1 in, 1 out]
          }
          frame #1 {
          }
        }
      }
      n224 = call <vilib>:"General Error Handler.vi"("error in (no error)"=w451) -> ()  [unwired: 1 in, 14 out]
      n225 = call "Variables.vi"("value"=string ?, "Tag in"=string ?, "Command"=T4 ?) -> ()  [unwired: 3 out]
      n226 = invoke class="VI" method="FP.Close"() -> ()  [unwired: 3 in, 3 out]
    }
  }
